vi "Pixy_COM-RIO.vi"() -> ()   [LabVIEW 2016]
uses:
  <vilib>/Rock Robotics/WPI/DriverStation/WPI_DriverStationRobotMode2.ctl
  <vilib>/Analysis/baseanly.llb/Mean (DBL).vi
  <vilib>/Instr/_visa.llb/VISA Configure Serial Port (Instr).vi
  Robot Global Data.vi
  <vilib>/Rock Robotics/Network Tables/NT Write Numeric Array.vi
  <vilib>/Analysis/NI_AALBase.lvlib
panel:
  out "Initialization error out":errorcluster
  out "Read error out":errorcluster
  in  "Display buffer size":u16=100 min=1
  out "Data display":string
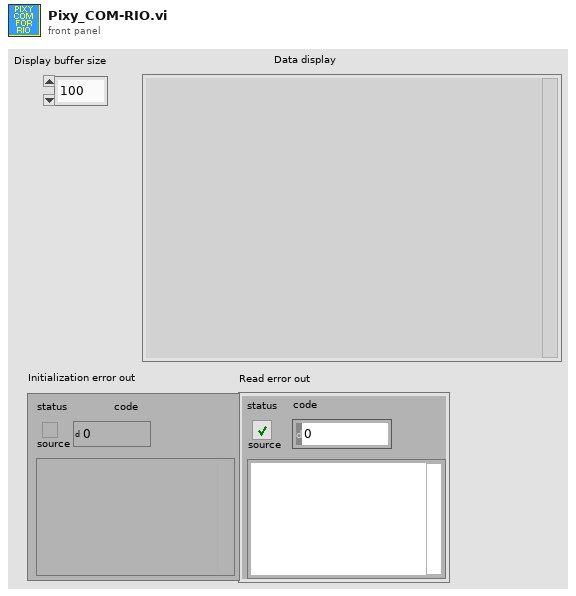
[diagram p1: front panel]
types:
  T1 = typedef "WPI_DriverStationRobotMode2.ctl" = enum16{"Autonomous Disabled", "Autonomous Enabled", "Teleop Disabled", "Teleop Enabled", "Disconnected", "Finish", "Test Disabled", "Test Enabled", "Emergency Stopped"}
  T2 = cluster{"buffer":string, "X":i32, "Y":i32, "Width":i32, "Height":i32, "Area":dbl}
  T3 = cluster{"Data out":cluster{"buffer":string, "X":i32, "Y":i32, "Width":i32, "Height":i32, "Area":dbl}, "Write Command?":bool, "Command":string}
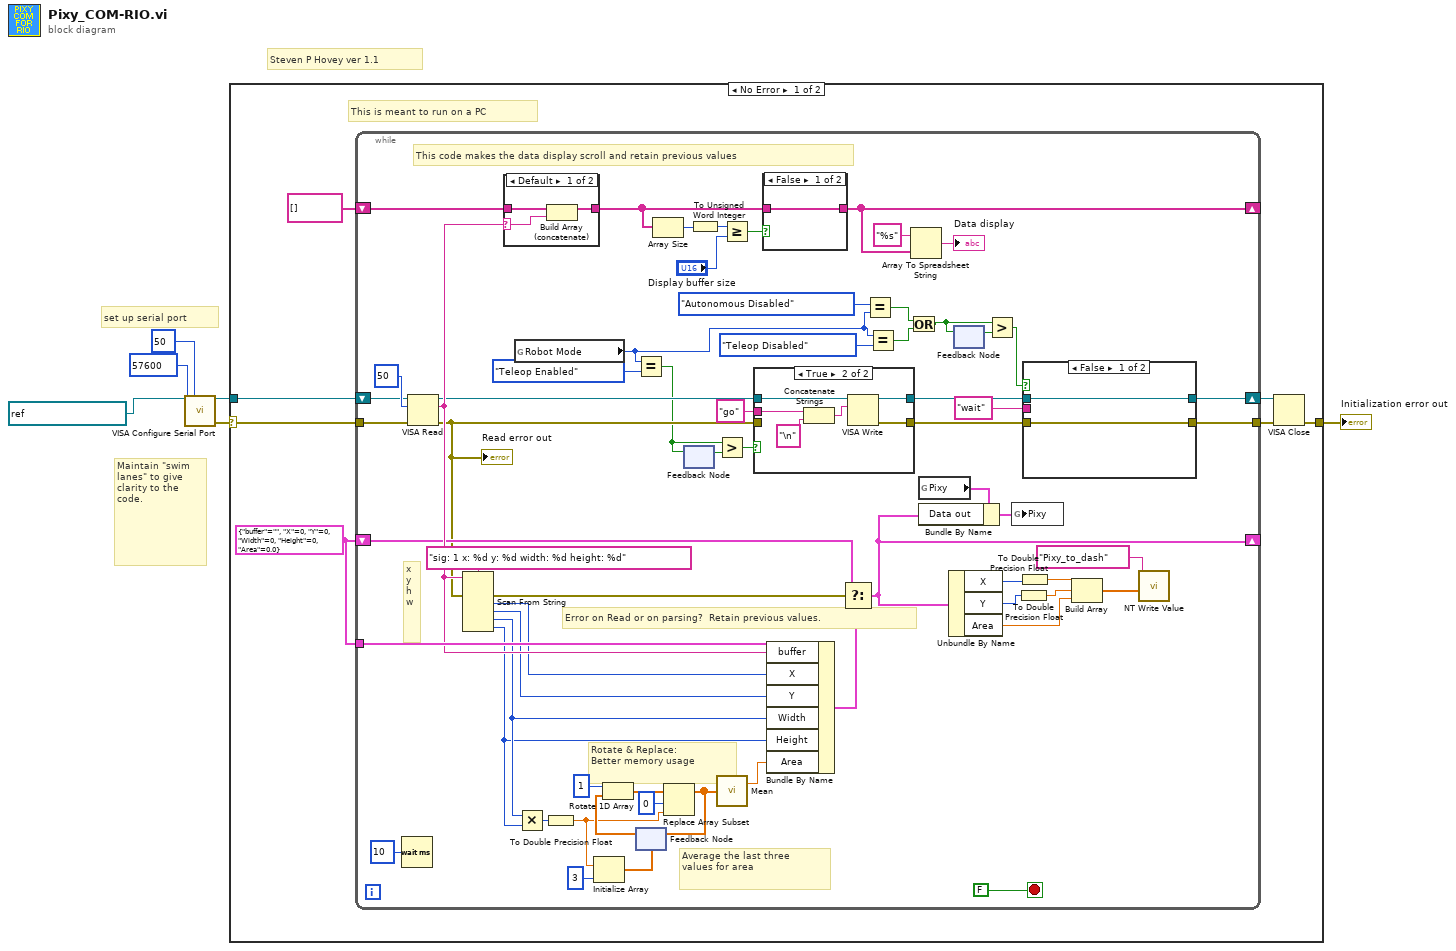
[diagram p0: block diagram]
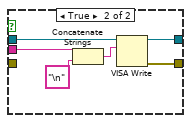
[diagram p2: hidden frame]
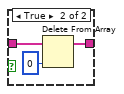
[diagram p4: hidden frame]
diagram:
  # "Maintain \"swim lanes\" to give clarity to the code."
  # "Steven P Hovey ver 1.1"
  # "set up serial port"
  n1 = call-poly "VISA Configure Serial Port"("VISA resource name"=refnum<visa-resource-name> "ASRL3::INSTR", "timeout (10sec)"=u32 50, "baud rate (9600)"=u32 57600) -> ("VISA resource name out"=w4:refnum<visa-resource-name>, "error out"=w2:errorcluster)  [unwired: 11 in]
  n2 = case shown="No Error" w2 {
    selector: w2 -> [w7 w102]
    tunnel: w4 -> [w13 _]
    tunnel: [w8 w102] -> w3
    frame No Error {
      w11 = T2 {"buffer"="", "X"=0, "Y"=0, "Width"=0, "Height"=0, "Area"=0.0}
      # "This is meant to run on a PC"
      n3 = while {
        shift-right: [w22] -> w10
        shift-left: w13 -> [w73]
        shift-right: [w41] -> _
        shift-left: w11 -> [w52]
        shift-right: [w45] -> _
        shift-left: string[] [] -> [w65]
        tunnel: w11 -> [w77]
        tunnel: w7 -> [w44]
        tunnel: [w23] -> w9
        stop <- FALSE ("stop") stop-if-true
        # "Error on Read or on parsing?  Retain previous values."
        # "Rotate & Replace:\nBetter memory usage"
        # "Average the last three\nvalues for area"
        # "This code makes the data display scroll and retain previous values"
        # "x\ny\nh\nw"
        n4 = Wait (ms)(milliseconds to wait=u32 10) -> ()  [unwired: 1 out]
        n5 = VISA Read(VISA resource name=w73, byte count=u32 50, error in (no error)=w44) -> (VISA resource name out=w67:refnum<visa-resource-name>, read buffer=w76:string, error out=w42:errorcluster)  [unwired: 1 out]
        "Read error out" <- w42
        n6 = Scan From String(format string="sig: 1 x: %d y: %d width: %d height: %d", input string=w76, error in=w42) -> (error out=w53:errorcluster, output 1=w58:i32, output 2=w57:i32, output 3=w56:i32, output 4=w55:i32)  [unwired: 5 in, 2 out]
        n7 = case shown="Default" w76 {
          selector: w76 -> [w86 _]
          tunnel: w65 -> [w87 w89]
          tunnel: [w88 w89] -> w46
          frame Default {
            n8 = Build Array (concatenate)(w87, w86) -> (w88:string[])
          }
          frame "" {
          }
        }
        n9 = global read "Robot Global Data.vi" "Robot Mode"() -> (w17:T1)
        n10 = Multiply(x=w56, y=w55) -> (x*y=w54:i32)
        n11 = To Double Precision Float(number=w54) -> (double precision float=w47:dbl)
        n12 = Initialize Array(w47, 3 ("dimension size")) -> (w70:dbl[])
        n13 = Equal?(x=w17, y=WPI_DriverStationRobotMode2."Teleop Enabled") -> (x = y?=w28:bool)
        n14 = feedback #1(w70) -> (w50:dbl[])
        n15 = Rotate 1D Array(1:w50, 2:1 ("n")) -> (0:w49:dbl[])
        n16 = Array Size(array=w46) -> (size(s)=w63:i32)
        n17 = Replace Array Subset(array=w49, new element=w47, index=0) -> (w69:dbl[])
        n18 = feedback-in #1(w69) -> ()
        n19 = feedback-in #2(w28) -> ()
        n20 = feedback #2() -> (w30:bool)  [unwired: 1 in]
        n21 = To Unsigned Word Integer(number=w63) -> (unsigned 16bit integer=w62:u16)
        n22 = Greater?(x=w28, y=w30) -> (0:w29:bool)
        n23 = call-poly <vilib>:"Mean.vi"("X"=w69) -> ("mean"=w72:dbl)  [unwired: 1 out]
        n24 = Greater Or Equal?(x=w62, y="Display buffer size") -> (x >= y?=w61:bool)
        n25 = case shown="True" w29 {
          tunnel: w67 -> [w95 w101]
          tunnel: [w95 w100] -> w25
          tunnel: "go" ("Command") -> [_ w99]
          tunnel: w42 -> [w94 _]
          tunnel: [w94 w98] -> w24
          frame False {
          }
          frame True {
            n26 = Concatenate Strings(w99, "\n") -> (w97:string)
            n27 = VISA Write(VISA resource name=w101, write buffer=w97) -> (VISA resource name out=w100:refnum<visa-resource-name>, error out=w98:errorcluster)  [unwired: 1 in, 1 out]
          }
        }
        n28 = case shown="False" w61 {
          tunnel: w46 -> [w90 w93]
          tunnel: [w90 w92] -> w45
          frame False {
          }
          frame True {
            n29 = Delete From Array(array=w93, index=0) -> (array with subset deleted=w92:string[])  [unwired: 1 in, 1 out]
          }
        }
        n30 = Bundle By Name(cluster=w77, "buffer"=w76, "X"=w58, "Y"=w57, "Width"=w56, "Height"=w55, "Area"=w72) -> (w51:T2)
        n31 = Select(t=w52, s=w53, f=w51) -> (s? t:f=w41:T2)
        n32 = Equal?(x=WPI_DriverStationRobotMode2."Autonomous Disabled" ("y"), y=w17) -> (x = y?=w15:bool)
        n33 = Equal?(x=w17, y=WPI_DriverStationRobotMode2."Teleop Disabled") -> (x = y?=w16:bool)
        n34 = Or(x=w15, y=w16) -> (x .or. y?=w14:bool)
        n35 = Array To Spreadsheet String(array=w45, 3:"%s" ("format string")) -> (spreadsheet string=→"Data display":string)  [unwired: 1 in]
        n36 = global read "Robot Global Data.vi" "Pixy"() -> (w40:T3)
        n37 = Bundle By Name(cluster=w40, "Data out"=w41) -> (w39:T3)
        n38 = Unbundle By Name(w41) -> ("X"=w38:i32, "Y"=w37:i32, "Area"=w36:dbl)
        n39 = feedback #3() -> (w20:bool)  [unwired: 1 in]
        n40 = feedback-in #3(w14) -> ()
        n41 = Greater?(x=w14, y=w20) -> (0:w19:bool)
        n42 = global write "Robot Global Data.vi" "Pixy"(w39) -> ()
        n43 = To Double Precision Float(number=w37) -> (double precision float=w35:dbl)
        n44 = To Double Precision Float(number=w38) -> (double precision float=w34:dbl)
        n45 = case shown="False" w19 {
          tunnel: w25 -> [w78 w83]
          tunnel: w24 -> [w79 _]
          tunnel: [w79 w81] -> w23
          tunnel: [w78 w82] -> w22
          tunnel: "wait" ("Command") -> [_ w80]
          frame False {
          }
          frame True {
            n46 = Concatenate Strings(w80, "\n") -> (w84:string)
            n47 = VISA Write(VISA resource name=w83, write buffer=w84) -> (VISA resource name out=w82:refnum<visa-resource-name>, error out=w81:errorcluster)  [unwired: 1 in, 1 out]
          }
        }
        n48 = Build Array(w34, w35, w36) -> (w33:dbl[])
        n49 = call-poly <vilib>:"NT Write Value.vi"("Numeric Array"=w33, "Name"="Pixy_to_dash") -> ()  [unwired: 9 in, 1 out]
      }
      n50 = VISA Close(VISA resource name=w10, error in (no error)=w9) -> (error out=w8:errorcluster)
    }
    frame Error {
    }
  }
  "Initialization error out" <- w3
